vi "_Update LDAC.vi"   [LabVIEW 2015]
uses:
  Instance           1 20Saved   _Update LDAC .vi
  <vilib>/rvi/eio/common/nirviEmuTemplateMethod_errors.vi
  <vilib>/eio/EIONode/EIONode.xnode
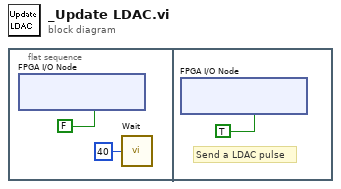
[diagram p0: block diagram]
diagram:
  n1 = flat-sequence {
    frame #0 {
      n2 = xnode "FPGA I/O Node"("Digtal IO/DIO63"=FALSE ("Digital Out")) -> ()  [unwired: 1 in, 1 out]
      n3 = call "Wait"("Count(Ticks)"=u8 40) -> ()  [unwired: 1 out]
    }
    frame #1 {
      # "Send a LDAC pulse"
      n4 = xnode "FPGA I/O Node"("Digtal IO/DIO63"=TRUE ("Digital Out")) -> ()  [unwired: 1 in, 1 out]
    }
  }
